vi "Result.Meas Status String to Status Enum.vi"(11 "Status Str":string) -> (3 "Status":T1 items=["LOG", "PASS", "FAIL", "ERROR"])   [LabVIEW 2024]
uses:
  Result.Measurement and Attribute Item Status.ctl
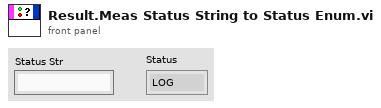
[diagram p1: front panel]
types:
  T1 = typedef "Result.Measurement and Attribute Item Status.ctl" = i32
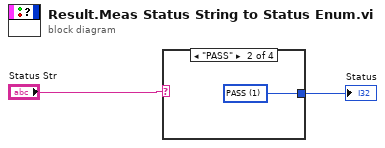
[diagram p0: block diagram]
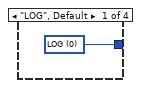
[diagram p2: hidden frame]
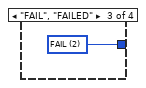
[diagram p3: hidden frame]
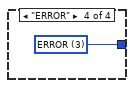
[diagram p4: hidden frame]
diagram:
  n1 = case shown="\"PASS\"" "Status Str" {
    tunnel: [w3 w4 w5 w6] -> w2
    frame "LOG", Default {
      w3 = T1 0 items=["LOG", "PASS", "FAIL", "ERROR"] ("Status")
    }
    frame "PASS" {
      w4 = T1 1 items=["LOG", "PASS", "FAIL", "ERROR"] ("Status")
    }
    frame "FAIL", "FAILED" {
      w5 = T1 2 items=["LOG", "PASS", "FAIL", "ERROR"] ("Status")
    }
    frame "ERROR" {
      w6 = T1 3 items=["LOG", "PASS", "FAIL", "ERROR"] ("Status")
    }
  }
  "Status" <- w2
